vi "Servo Pulse Gen._2.vi"() -> ()   [LabVIEW 2020]
uses:
  LCD Pressing Servo.ctl
  Galobal variable_TI.vi
  Project Setup/Globle Variable/GR_Servo.vi
panel:
  out "Servo _Motor2":T1
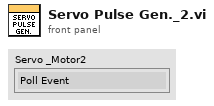
[diagram p1: front panel]
types:
  T1 = typedef "LCD Pressing Servo.ctl" = enum16{"Poll Event", "LCD  Press ServoCMD", "LCD Press Servo Home", "Exit"}
  T2 = cluster{"Emergency":bool, "Air Pressure":bool, "Saftey Sensor":bool, "Slide Servo  fault":bool, "LCD Pressing  Servo  fault":bool, "Reset":bool}
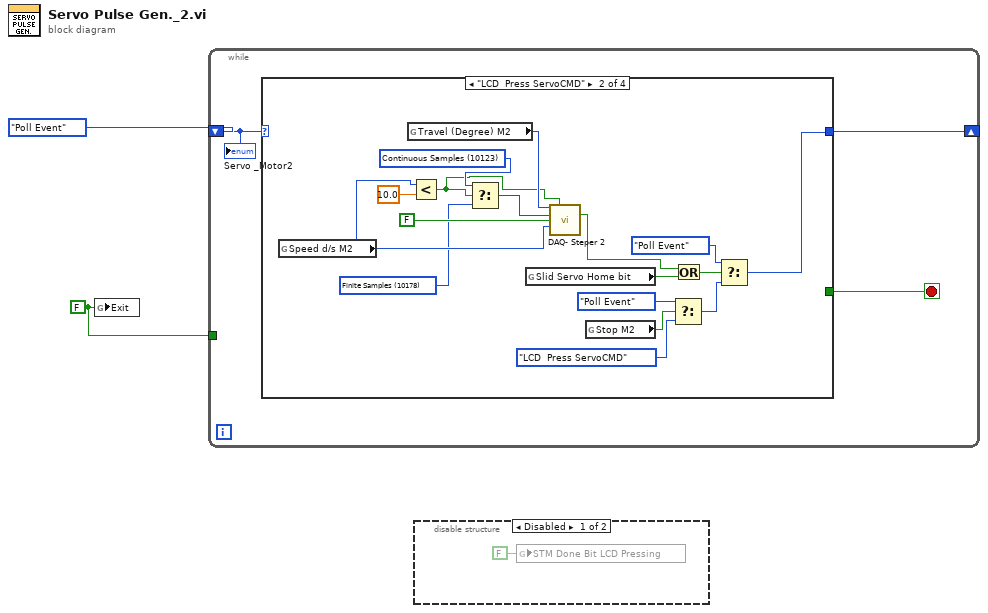
[diagram p0: block diagram]
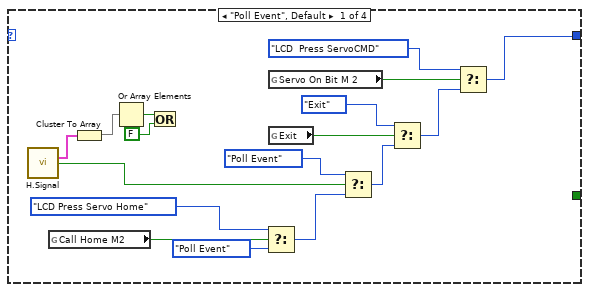
[diagram p3: hidden frame]
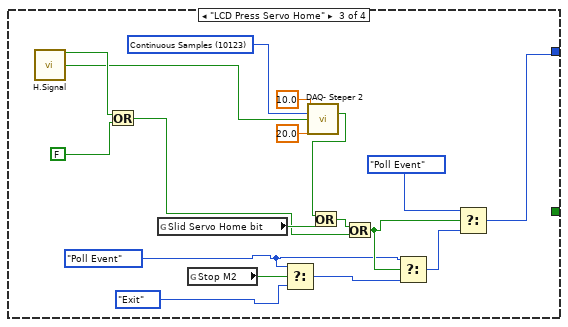
[diagram p4: hidden frame]
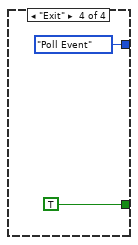
[diagram p5: hidden frame]
diagram:
  w1 = FALSE ("Exit")
  n1 = global write "Galobal variable_TI.vi" "Exit"(w1) -> ()
  n2 = while {
    shift-right: [w4] -> _
    shift-left: LCD_Pressing_Servo."Poll Event" ("Servo _Motor2") -> [w5]
    tunnel: w1 -> [_]
    stop <- w3 stop-if-true
    n3 = case shown="\"LCD  Press ServoCMD\"" w5 {
      tunnel: [w11 w30 w41 LCD_Pressing_Servo."Poll Event" ("f")] -> w4
      tunnel: [_ _ _ TRUE] -> w3
      frame "Poll Event", Default {
        n4 = call "H.Signal.vi"() -> ("H.Signal"=w9:T2, "LCD Pressing servo home RS"=w10:bool)  [unwired: 10 in, 4 out]
        n5 = global read "Galobal variable_TI.vi" "Call Home M2"() -> (w16:bool)
        n6 = Cluster To Array(cluster=w9) -> (array=w8:bool[])
        n7 = Or Array Elements(Boolean array=w8) -> (logical OR=w7:bool)
        n8 = Or(x=w7, y=FALSE) -> ()  [unwired: 1 out]
        n9 = Select(t=LCD_Pressing_Servo."LCD Press Servo Home" ("Servo _Motor2"), s=w16, f=LCD_Pressing_Servo."Poll Event") -> (s? t:f=w13:T1)
        n10 = global read "GR_Servo.vi" "Servo On Bit M 2"() -> (w21:bool)
        n11 = global read "Galobal variable_TI.vi" "Exit"() -> (w20:bool)
        n12 = Select(t=LCD_Pressing_Servo."Poll Event" ("Servo _Motor2"), s=w10, f=w13) -> (s? t:f=w12:T1)
        n13 = Select(t=LCD_Pressing_Servo."Exit" ("Servo _Motor2"), s=w20, f=w12) -> (s? t:f=w18:T1)
        n14 = Select(t=LCD_Pressing_Servo."LCD  Press ServoCMD" ("Servo _Motor2"), s=w21, f=w18) -> (s? t:f=w11:T1)
      }
      frame "LCD  Press ServoCMD" {
        w26 = 10178 items=["Finite Samples"=10178, "Continuous Samples"=10123, "Hardware Timed Single Point"=12522] ("Mode")
        w25 = 10123 items=["Finite Samples"=10178, "Continuous Samples"=10123, "Hardware Timed Single Point"=12522] ("Mode")
        n15 = global read "GR_Servo.vi" "Speed d/s M2"() -> (w27:i32)
        n16 = global read "GR_Servo.vi" "Travel (Degree) M2"() -> (w39:i32)
        n17 = Less?(x=w27, y=10.0) -> (x < y?=w23:bool)
        n18 = Select(t=w25, s=w23, f=w26) -> (s? t:f=w24:i32)
        n19 = global read "Galobal variable_TI.vi" "Slid Servo Home bit"() -> (w31:bool)
        n20 = call "DAQ- Steper 2.vi"("Travel (Degree)"=w39, "Loda based"=w23, "Mode"=w24, "Home Done"=FALSE, "Speed d/s"=w27) -> ("Task Done Bit"=w29:bool)  [unwired: 9 in, 1 out]
        n21 = global read "Galobal variable_TI.vi" "Stop M2"() -> (w33:bool)
        n22 = Select(t=LCD_Pressing_Servo."Poll Event" ("Servo _Motor2"), s=w33, f=LCD_Pressing_Servo."LCD  Press ServoCMD" ("Servo _Motor2")) -> (s? t:f=w34:T1)
        n23 = Or(x=w29, y=w31) -> (x .or. y?=w32:bool)
        n24 = Select(t=LCD_Pressing_Servo."Poll Event" ("Servo _Motor2"), s=w32, f=w34) -> (s? t:f=w30:T1)
      }
      frame "LCD Press Servo Home" {
        w44 = LCD_Pressing_Servo."Poll Event" ("Servo _Motor2")
        w57 = 10123 items=["Finite Samples"=10178, "Continuous Samples"=10123, "Hardware Timed Single Point"=12522] ("Mode")
        n25 = call "H.Signal.vi"() -> ("Slide servo home RS"=w53:bool, "LCD Pressing servo home RS"=w52:bool)  [unwired: 10 in, 4 out]
        n26 = Or(x=w53, y=FALSE) -> (x .or. y?=w40:bool)
        n27 = global read "Galobal variable_TI.vi" "Slid Servo Home bit"() -> (w51:bool)
        n28 = global read "Galobal variable_TI.vi" "Stop M2"() -> (w49:bool)
        n29 = Select(t=w44, s=w49, f=LCD_Pressing_Servo."Exit" ("Servo _Motor2")) -> (s? t:f=w47:T1)
        n30 = call "DAQ- Steper 2.vi"("Travel (Degree)"=10.0, "Mode"=w57, "Home Done"=w52, "Speed d/s"=20.0) -> ("Task Done Bit"=w42:bool)  [unwired: 10 in, 1 out]
        n31 = Or(x=w42, y=w51) -> (x .or. y?=w50:bool)
        n32 = Or(x=w50, y=w40) -> (x .or. y?=w48:bool)
        n33 = Select(t=w44, s=w48, f=w47) -> (s? t:f=w46:T1)
        n34 = Select(t=LCD_Pressing_Servo."Poll Event" ("Servo _Motor2"), s=w48, f=w46) -> (s? t:f=w41:T1)
      }
      frame "Exit" {
      }
    }
    "Servo _Motor2" <- w5
  }
  n35 = disable-structure shown="Disabled" {
    frame Disabled {
      n36 = global write "GR_Servo.vi" "STM Done Bit LCD Pressing"(FALSE ("STM Done Bit LCD Pressing")) -> ()
    }
    frame Enabled {
    }
  }
